vi "fit.vi"(8 "error in (no error)":errorcluster caption="entrée d'erreur (pas d'erreur)", 11 "Tree.lvclass 2":refnum<class "Tree.lvclass">) -> (0 "error out":errorcluster caption="sortie d'erreur", 3 "Tree.lvclass":refnum<class "Tree.lvclass">)   [LabVIEW 2020, in "Tree.lvclass"]
doc: "Build a decision tree regressor from the training set (X, y).\n\n Parameters\n ----------\n X : {array-like, sparse matrix} of shape (n_samples, n_features)\n The training input samples. Internally, it will be converted to\n ``dtype=np.float32`` and if a sparse matrix is provided\n to a sparse ``csc_matrix``.\n\n y : array-like of shape (n_samples,) or (n_samples, n_outputs)\n The target values (real numbers). Use ``dtype=np.float64`` and\n ``order='C'`` for maximum efficiency.\n\n sample_weight : array-like of shape (n_samples,), default=None\n Sample weights. If None, then samples are equally weighted. Splits\n that would create child nodes with net zero or negative weight are\n ignored while searching for a split in each node.\n\n check_input : bool, default=True\n Allow to bypass several input checking.\n Don't use this parameter unless you know what you do.\n\n Returns\n -------\n self : DecisionTreeRegressor\n Fitted estimator."
uses:
  Tree.lvclass
  C:/Users/cipop/TDF Dropbox/2_Technologies de France/1 - Services et Etudes/PLAIY/2 - DEV/PLAIYLAB/code/Python/Python.lvclass
  C:/Users/cipop/TDF Dropbox/2_Technologies de France/1 - Services et Etudes/PLAIY/2 - DEV/PLAIYLAB/code/Model/Model.lvclass
  Tree.lvclass/Tree.ctl
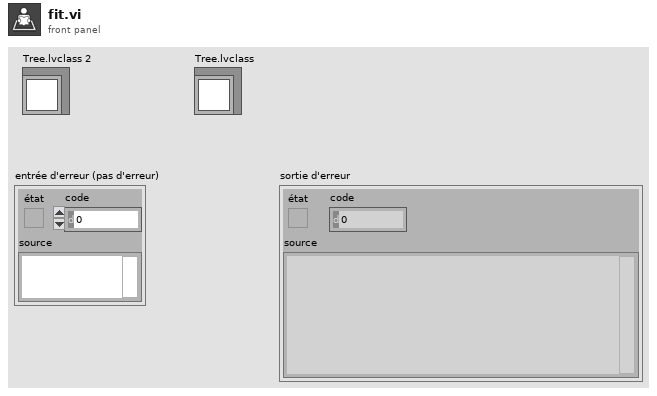
[diagram p1: front panel]
types:
  T1 = typedef "data.ctl" = cluster{"name":string, "X":dbl[][]}
  T2 = typedef "tree_data.ctl" = cluster{"y":dbl[][], "sample_weight":dbl[], "check_input":bool}
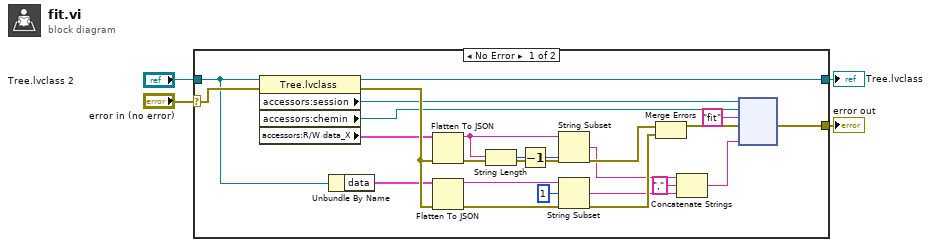
[diagram p0: block diagram]
diagram:
  n1 = case shown="No Error" "error in (no error)" {
    selector: "error in (no error)" -> [w24 w28]
    tunnel: [w25 w28] -> w3
    tunnel: [w7 w27] -> w1
    tunnel: "Tree.lvclass 2" -> [w6 w27]
    frame No Error {
      n2 = property class="Tree.lvclass"(reference=w6, error in=w24) -> (reference out=w7:refnum<class "Tree.lvclass">, error out=w20:errorcluster, "accessors:session"=w10:refnum<k35>, "accessors:chemin"=w9:path, "accessors:R/W data_X"=w11:T1)
      n3 = Unbundle By Name(w6) -> ("data"=w5:T2)
      n4 = Flatten To JSON(anything=w11, error in (no error)=w20) -> (JSON string=w21:string, 11:w16:errorcluster)  [unwired: 1 in]
      n5 = Flatten To JSON(anything=w5, error in (no error)=w20) -> (JSON string=w18:string, 11:w17:errorcluster)  [unwired: 1 in]
      n6 = String Length(string=w21) -> (length=w23:i32)
      n7 = Decrement(x=w23) -> (x-1=w22:i32)
      n8 = String Subset(string=w21, length (rest)=w22) -> (substring=w14:string)  [unwired: 1 in]
      n9 = String Subset(string=w18, offset (0)=1) -> (substring=w13:string)  [unwired: 1 in]
      n10 = Merge Errors(w16, w17) -> (w8:errorcluster)
      n11 = Concatenate Strings(w14, "," ("string"), w13) -> (w12:string)
      n12 = node(w10, w9, "fit" ("nom de la fonction"), w8, w12) -> (w25:errorcluster)  [unwired: 3 in, 3 out]
    }
    frame Error {
    }
  }
  "error out" <- w3
  "Tree.lvclass" <- w1
